vi "Savitsky Golay Filter (single).vi"(6 "Side Points Unit (points)":enum16{"Points", "Data"}(ring), 8 "error in (no error)":errorcluster, 10 "side points":dbl, 11 "XY-data":cluster{"X-array":dbl[], "Y-array":dbl[]}) -> (0 "error out":errorcluster, 3 "XY-data out":cluster{"X-array":dbl[], "Y-array":dbl[]} {"Y-array" format="%.2p"; "X-array" format="%.2p"})   [LabVIEW 2016, in "xy_utilities.lvlib"]
doc: "Filter <b>XY-data</b>'s Y-Array with a Savitsky-Golay FIR smoothing filter.\n\n<b>side points</b> specifies the number of data points to each side of the current data point to use for the least squares minimization. side points*2 + 1 is the length of the moving window, which must be greater than the polynomial order.\n\nWire data to the data input to determine the polymorphic instance to use or manually select the instance."
uses:
  xy_utilities.lvlib
  <vilib>/Analysis/3filter.llb/Savitzky-Golay Filter (DBL).vi
  Private/X Array Range to Index.vi
  <vilib>/Analysis/NI_AALBase.lvlib
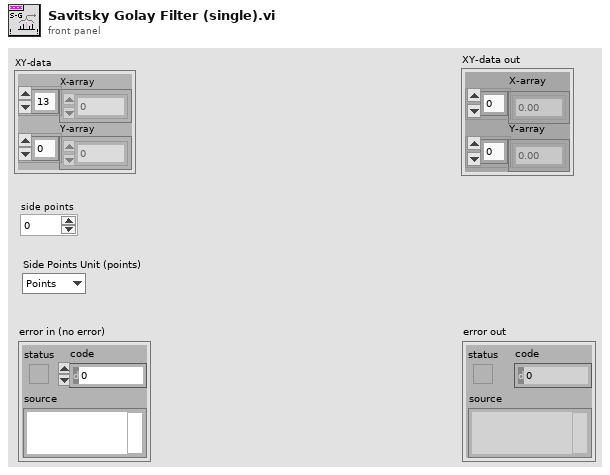
[diagram p1: front panel]
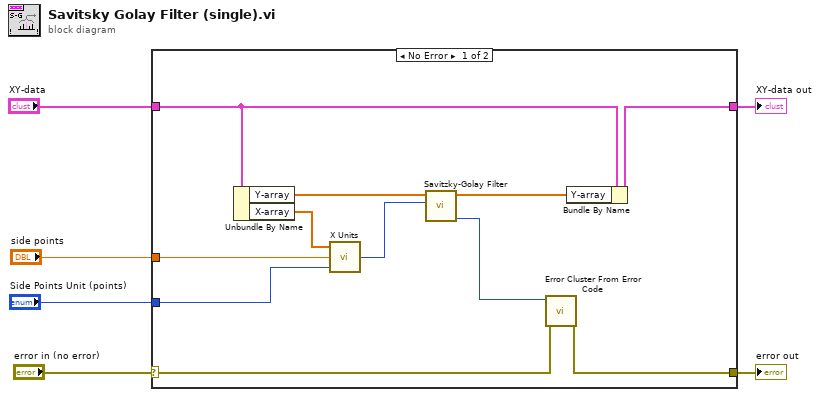
[diagram p0: block diagram]
diagram:
  n1 = case shown="No Error" "error in (no error)" {
    selector: "error in (no error)" -> [w12 w19]
    tunnel: [w11 w19] -> w5
    tunnel: "XY-data" -> [w16 w18]
    tunnel: [w17 w18] -> w3
    tunnel: "side points" -> [w9 _]
    tunnel: "Side Points Unit (points)" -> [w7 _]
    frame No Error {
      n2 = Unbundle By Name(w16) -> ("Y-array"=w15:dbl[], "X-array"=w10:dbl[])
      n3 = call "X Units.vi"("Interval Units (points)"=w7, "Interval (h)"=w9, "X-array"=w10) -> ("h (points)"=w8:i32)
      n4 = call-poly <vilib>:"Savitzky-Golay Filter.vi"("side points"=w8, "X"=w15) -> ("error"=w13:i32, "Filtered X"=w14:dbl[])  [unwired: 8 in]
      n5 = call <vilib>:"Error Cluster From Error Code.vi"("error in (no error)"=w12, "error code (0)"=w13) -> ("error out"=w11:errorcluster)  [unwired: 7 in]
      n6 = Bundle By Name(cluster=w16, "Y-array"=w14) -> (w17:cluster{"X-array":dbl[], "Y-array":dbl[]})
    }
    frame Error {
    }
  }
  "error out" <- w5
  "XY-data out" <- w3
